vi "Test Connected Device.vi"(8 "error in (no error)":errorcluster, 11 "Read Buffer":string) -> (0 "error out":errorcluster, 2 "Connected":bool, 3 "Device Info":string[](array[string]))   [LabVIEW 2025]
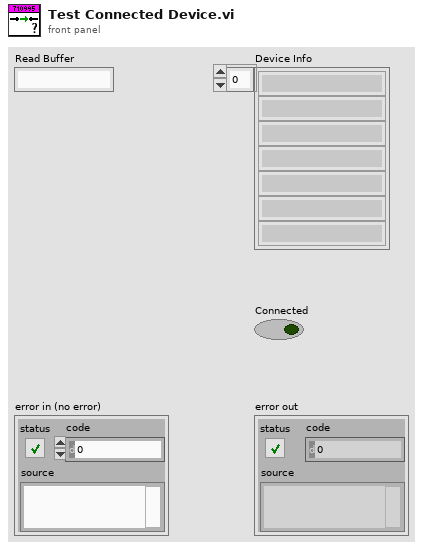
[diagram p1: front panel]
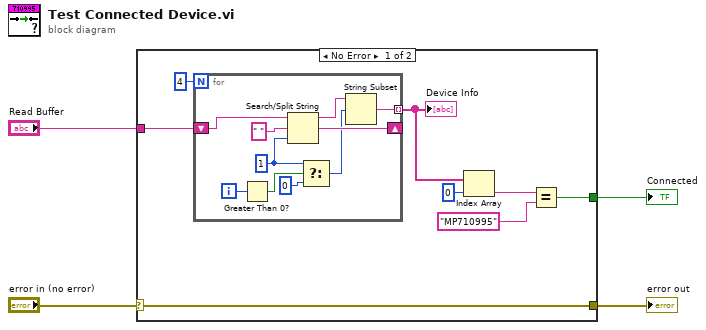
[diagram p0: block diagram]
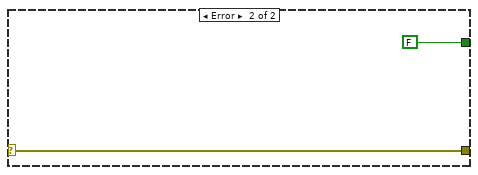
[diagram p2: hidden frame]
diagram:
  n1 = case shown="No Error" "error in (no error)" {
    selector: "error in (no error)" -> [w5 w24]
    tunnel: "Read Buffer" -> [w12 _]
    tunnel: [w6 FALSE] -> w2
    tunnel: [w5 w24] -> w4
    frame No Error {
      n2 = for {
        N: 4 -> [_]
        shift-right: [w21] -> _
        shift-left: w12 -> [w22]
        tunnel: [w14] -> w7 mode=indexing
        i -> [w20]
        w18 = 1 ("offset (0)")
        n3 = Greater Than 0?(x=w20) -> (x > 0?=w19:bool)
        n4 = Search/Split String(string=w22, search string/char (-)=" ", offset (0)=w18) -> (substring before match=w15:string, match + rest of string=w21:string)  [unwired: 1 out]
        n5 = Select(t=w18, s=w19, f=0) -> (s? t:f=w16:i32)
        n6 = String Subset(string=w15, offset (0)=w16) -> (substring=w14:string)  [unwired: 1 in]
      }
      "Device Info" <- w7
      n7 = Index Array(array=w7, index=0) -> (element=w9:string)
      n8 = Equal?(x=w9, y="MP710995") -> (x = y?=w6:bool)
    }
    frame Error {
    }
  }
  "error out" <- w4
  "Connected" <- w2
